vi "Get Item Property Pack Variant.vi"(6 "Default Value":variant, 8 "error in (no error)":errorcluster, 10 "Property Name":string, 11 "CDBase":refnum<k39>) -> (0 "error out":errorcluster, 1 "Found?":bool, 2 "Variant":variant, 3 "CDBase":refnum<k39>)   [LabVIEW 2026, in "Custom Devices Storage.lvlib"]
uses:
  Custom Devices Storage.lvlib
  C:/Users/Administrator/Desktop/Jatin/All DNC DLLs/NationalInstruments.VeriStand.SystemDefinitionAPI.dll
  Jatin/All DNC DLLs/NationalInstruments.VeriStand.SystemDefinitionAPI.dll
  C:/Users/Administrator/Desktop/Jatin/All DNC DLLs/NationalInstruments.VeriStand.SystemStorage.dll
  Jatin/All DNC DLLs/NationalInstruments.VeriStand.SystemStorage.dll
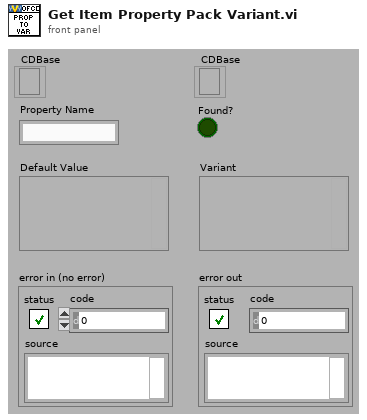
[diagram p1: front panel]
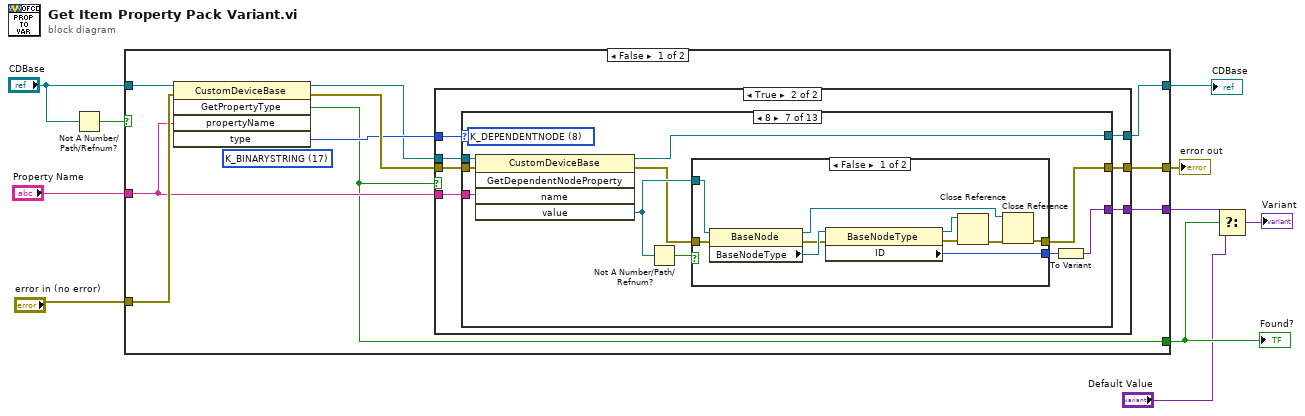
[diagram p0: block diagram]
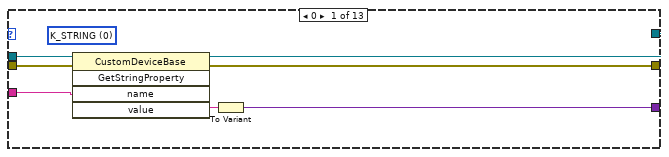
[diagram p3: hidden frame]
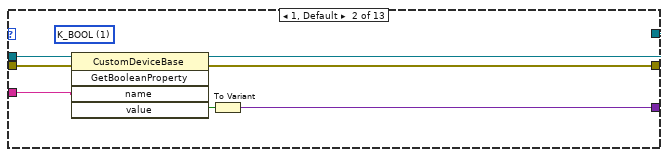
[diagram p4: hidden frame]
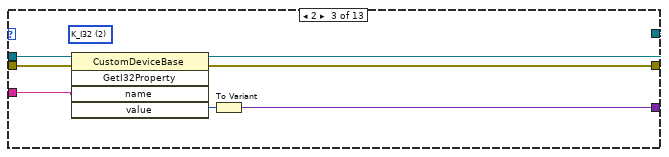
[diagram p5: hidden frame]
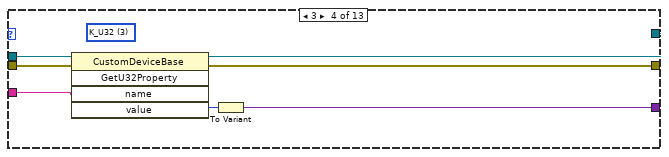
[diagram p6: hidden frame]
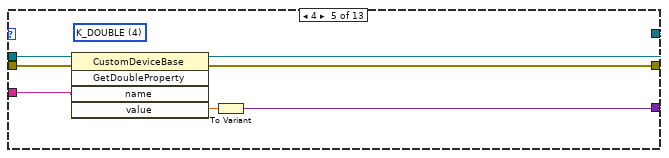
[diagram p7: hidden frame]
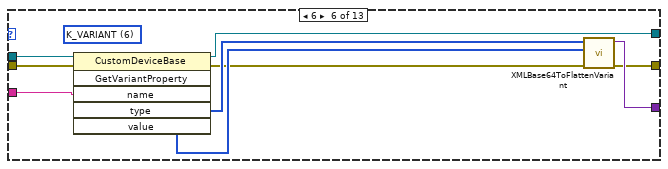
[diagram p8: hidden frame]
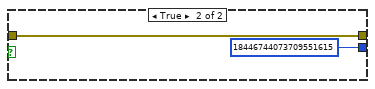
[diagram p9: hidden frame]
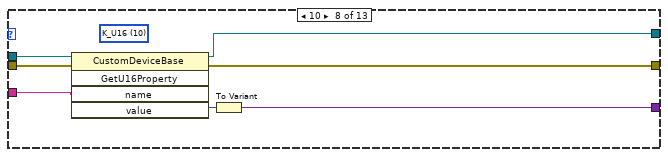
[diagram p10: hidden frame]
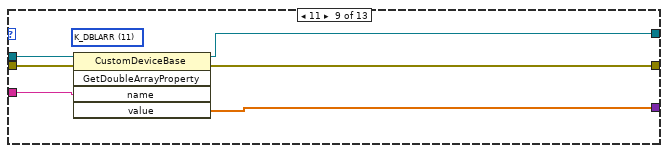
[diagram p11: hidden frame]
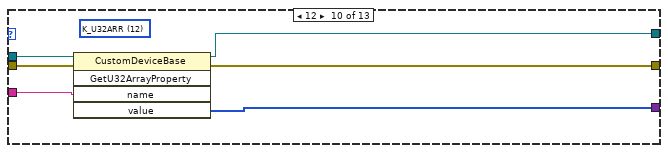
[diagram p12: hidden frame]
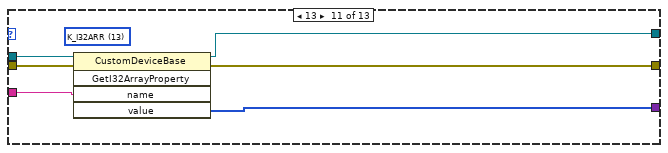
[diagram p13: hidden frame]
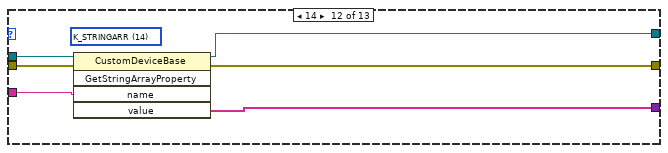
[diagram p14: hidden frame]
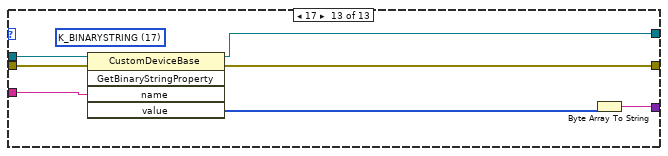
[diagram p15: hidden frame]
diagram:
  n1 = Not A Number/Path/Refnum?(number/path/refnum="CDBase") -> (NaN/Path/Refnum?=w10:bool)
  n2 = case shown="False" w10 {
    tunnel: "Property Name" -> [w15 _]
    tunnel: "CDBase" -> [w20 w135]
    tunnel: "error in (no error)" -> [w19 w134]
    tunnel: [w14 _] -> w6
    tunnel: [w13 _] -> w5
    tunnel: [w12 w135] -> w2
    tunnel: [w11 w134] -> w1
    frame False {
      (unwired) 17 items=["K_STRING", "K_BOOL", "K_I32", "K_U32", "K_DOUBLE", "K_U64", "K_VARIANT", "K_DEPENDENTFILE", "K_DEPENDENTNODE", "K_DATASOURCENODE", "K_U16", "K_DBLARR", "K_U32ARR", "K_I32ARR", "K_STRINGARR", "K_DICTIONARY", "K_DICTIONARYARR", "K_BINARYSTRING"] ("type")
      n3 = invoke class="CustomDeviceBase" method="GetPropertyType"(reference=w20, error in=w19, "propertyName"=w15) -> (reference out=w16:refnum<k39>, error out=w18:errorcluster, "GetPropertyType"=w14:bool, "type"=w17:i32)  [unwired: 2 in, 1 out]
      n4 = case shown="True" w14 {
        tunnel: [w21 w29] -> w12
        tunnel: [w22 w28] -> w11
        tunnel: [_ w27] -> w13
        tunnel: w18 -> [w22 w26]
        tunnel: w17 -> [_ w25]
        tunnel: w16 -> [w21 w24]
        tunnel: w15 -> [_ w23]
        frame False {
        }
        frame True {
          n5 = case shown="8" w25 {
            tunnel: [w36 w43 w50 w57 w64 w73 w80 w102 w108 w114 w120 w122 w127] -> w29
            tunnel: w26 -> [w35 w42 w49 w56 w63 w72 w83 w101 w107 w113 w119 w126 w132]
            tunnel: [w34 w41 w48 w55 w62 w65 w75 w100 w106 w112 w118 w125 w128] -> w28
            tunnel: [w32 w39 w46 w53 w60 w66 w79 w98 w105 w111 w117 w124 w129] -> w27
            tunnel: w24 -> [w30 w38 w44 w51 w58 w71 w82 w97 w103 w110 w116 w121 w133]
            tunnel: w23 -> [w31 w37 w45 w52 w59 w70 w81 w96 w104 w109 w115 w123 w131]
            frame 0 {
              (unwired) 0 items=["K_STRING", "K_BOOL", "K_I32", "K_U32", "K_DOUBLE", "K_U64", "K_VARIANT", "K_DEPENDENTFILE", "K_DEPENDENTNODE", "K_DATASOURCENODE", "K_U16", "K_DBLARR", "K_U32ARR", "K_I32ARR", "K_STRINGARR", "K_DICTIONARY", "K_DICTIONARYARR"] ("type")
              n6 = invoke class="CustomDeviceBase" method="GetStringProperty"(reference=w30, error in=w35, "name"=w31) -> (reference out=w36:refnum<k39>, error out=w34:errorcluster, "value"=w33:string)  [unwired: 2 in, 2 out]
              n7 = To Variant(anything=w33) -> (Variant=w32:variant)
            }
            frame 1, Default {
              (unwired) 1 items=["K_STRING", "K_BOOL", "K_I32", "K_U32", "K_DOUBLE", "K_U64", "K_VARIANT", "K_DEPENDENTFILE", "K_DEPENDENTNODE", "K_DATASOURCENODE", "K_U16", "K_DBLARR", "K_U32ARR", "K_I32ARR", "K_STRINGARR", "K_DICTIONARY", "K_DICTIONARYARR"] ("type")
              n8 = invoke class="CustomDeviceBase" method="GetBooleanProperty"(reference=w38, error in=w42, "name"=w37) -> (reference out=w43:refnum<k39>, error out=w41:errorcluster, "value"=w40:bool)  [unwired: 2 in, 2 out]
              n9 = To Variant(anything=w40) -> (Variant=w39:variant)
            }
            frame 2 {
              (unwired) 2 items=["K_STRING", "K_BOOL", "K_I32", "K_U32", "K_DOUBLE", "K_U64", "K_VARIANT", "K_DEPENDENTFILE", "K_DEPENDENTNODE", "K_DATASOURCENODE", "K_U16", "K_DBLARR", "K_U32ARR", "K_I32ARR", "K_STRINGARR", "K_DICTIONARY", "K_DICTIONARYARR"] ("type")
              n10 = invoke class="CustomDeviceBase" method="GetI32Property"(reference=w44, error in=w49, "name"=w45) -> (reference out=w50:refnum<k39>, error out=w48:errorcluster, "value"=w47:i32)  [unwired: 2 in, 2 out]
              n11 = To Variant(anything=w47) -> (Variant=w46:variant)
            }
            frame 3 {
              (unwired) 3 items=["K_STRING", "K_BOOL", "K_I32", "K_U32", "K_DOUBLE", "K_U64", "K_VARIANT", "K_DEPENDENTFILE", "K_DEPENDENTNODE", "K_DATASOURCENODE", "K_U16", "K_DBLARR", "K_U32ARR", "K_I32ARR", "K_STRINGARR", "K_DICTIONARY", "K_DICTIONARYARR"] ("type")
              n12 = invoke class="CustomDeviceBase" method="GetU32Property"(reference=w51, error in=w56, "name"=w52) -> (reference out=w57:refnum<k39>, error out=w55:errorcluster, "value"=w54:u32)  [unwired: 2 in, 2 out]
              n13 = To Variant(anything=w54) -> (Variant=w53:variant)
            }
            frame 4 {
              (unwired) 4 items=["K_STRING", "K_BOOL", "K_I32", "K_U32", "K_DOUBLE", "K_U64", "K_VARIANT", "K_DEPENDENTFILE", "K_DEPENDENTNODE", "K_DATASOURCENODE", "K_U16", "K_DBLARR", "K_U32ARR", "K_I32ARR", "K_STRINGARR", "K_DICTIONARY", "K_DICTIONARYARR"] ("type")
              n14 = invoke class="CustomDeviceBase" method="GetDoubleProperty"(reference=w58, error in=w63, "name"=w59) -> (reference out=w64:refnum<k39>, error out=w62:errorcluster, "value"=w61:dbl)  [unwired: 2 in, 2 out]
              n15 = To Variant(anything=w61) -> (Variant=w60:variant)
            }
            frame 6 {
              (unwired) 6 items=["K_STRING", "K_BOOL", "K_I32", "K_U32", "K_DOUBLE", "K_U64", "K_VARIANT", "K_DEPENDENTFILE", "K_DEPENDENTNODE", "K_DATASOURCENODE", "K_U16", "K_DBLARR", "K_U32ARR", "K_I32ARR", "K_STRINGARR", "K_DICTIONARY", "K_DICTIONARYARR"] ("type")
              n16 = invoke class="CustomDeviceBase" method="GetVariantProperty"(reference=w71, error in=w72, "name"=w70) -> (reference out=w73:refnum<k39>, error out=w67:errorcluster, "type"=w69:u8[], "value"=w68:u8[])  [unwired: 3 in, 2 out]
              n17 = call "XMLBase64ToFlattenVariant.vi"("error in (no error)"=w67, "Data"=w68, "Type array"=w69) -> ("error out"=w65:errorcluster, "Variant"=w66:variant)  [unwired: 7 in]
            }
            frame 8 {
              (unwired) 8 items=["K_STRING", "K_BOOL", "K_I32", "K_U32", "K_DOUBLE", "K_U64", "K_VARIANT", "K_DEPENDENTFILE", "K_DEPENDENTNODE", "K_DATASOURCENODE", "K_U16", "K_DBLARR", "K_U32ARR", "K_I32ARR", "K_STRINGARR", "K_DICTIONARY", "K_DICTIONARYARR"] ("type")
              n18 = invoke class="CustomDeviceBase" method="GetDependentNodeProperty"(reference=w82, error in=w83, "name"=w81) -> (reference out=w80:refnum<k39>, error out=w76:errorcluster, "value"=w77:refnum<k39>)  [unwired: 2 in, 2 out]
              n19 = Not A Number/Path/Refnum?(number/path/refnum=w77) -> (NaN/Path/Refnum?=w78:bool)
              n20 = case shown="False" w78 {
                tunnel: w76 -> [w93 w95]
                tunnel: [w87 w95] -> w75
                tunnel: w77 -> [w92 _]
                tunnel: [w90 u64 18446744073709551615 ("NodePtr")] -> w74
                frame False {
                  n21 = property class="BaseNode"(reference=w92, error in=w93) -> (reference out=w85:refnum<k39>, error out=w84:errorcluster, "BaseNodeType"=w91:refnum<k39>)
                  n22 = property class="BaseNodeType"(reference=w91, error in=w84) -> (reference out=w86:refnum<k39>, error out=w89:errorcluster, "ID"=w90:u64)
                  n23 = Close Reference(reference=w86, error in (no error)=w89) -> (error out=w88:errorcluster)
                  n24 = Close Reference(reference=w85, error in (no error)=w88) -> (error out=w87:errorcluster)
                }
                frame True {
                }
              }
              n25 = To Variant(anything=w74) -> (Variant=w79:variant)
            }
            frame 10 {
              (unwired) 10 items=["K_STRING", "K_BOOL", "K_I32", "K_U32", "K_DOUBLE", "K_U64", "K_VARIANT", "K_DEPENDENTFILE", "K_DEPENDENTNODE", "K_DATASOURCENODE", "K_U16", "K_DBLARR", "K_U32ARR", "K_I32ARR", "K_STRINGARR", "K_DICTIONARY", "K_DICTIONARYARR"] ("type")
              n26 = invoke class="CustomDeviceBase" method="GetU16Property"(reference=w97, error in=w101, "name"=w96) -> (reference out=w102:refnum<k39>, error out=w100:errorcluster, "value"=w99:u16)  [unwired: 2 in, 2 out]
              n27 = To Variant(anything=w99) -> (Variant=w98:variant)
            }
            frame 11 {
              (unwired) 11 items=["K_STRING", "K_BOOL", "K_I32", "K_U32", "K_DOUBLE", "K_U64", "K_VARIANT", "K_DEPENDENTFILE", "K_DEPENDENTNODE", "K_DATASOURCENODE", "K_U16", "K_DBLARR", "K_U32ARR", "K_I32ARR", "K_STRINGARR", "K_DICTIONARY", "K_DICTIONARYARR"] ("type")
              n28 = invoke class="CustomDeviceBase" method="GetDoubleArrayProperty"(reference=w103, error in=w107, "name"=w104) -> (reference out=w108:refnum<k39>, error out=w106:errorcluster, "value"=w105:dbl[])  [unwired: 2 in, 2 out]
            }
            frame 12 {
              (unwired) 12 items=["K_STRING", "K_BOOL", "K_I32", "K_U32", "K_DOUBLE", "K_U64", "K_VARIANT", "K_DEPENDENTFILE", "K_DEPENDENTNODE", "K_DATASOURCENODE", "K_U16", "K_DBLARR", "K_U32ARR", "K_I32ARR", "K_STRINGARR", "K_DICTIONARY", "K_DICTIONARYARR"] ("type")
              n29 = invoke class="CustomDeviceBase" method="GetU32ArrayProperty"(reference=w110, error in=w113, "name"=w109) -> (reference out=w114:refnum<k39>, error out=w112:errorcluster, "value"=w111:u32[])  [unwired: 2 in, 2 out]
            }
            frame 13 {
              (unwired) 13 items=["K_STRING", "K_BOOL", "K_I32", "K_U32", "K_DOUBLE", "K_U64", "K_VARIANT", "K_DEPENDENTFILE", "K_DEPENDENTNODE", "K_DATASOURCENODE", "K_U16", "K_DBLARR", "K_U32ARR", "K_I32ARR", "K_STRINGARR", "K_DICTIONARY", "K_DICTIONARYARR"] ("type")
              n30 = invoke class="CustomDeviceBase" method="GetI32ArrayProperty"(reference=w116, error in=w119, "name"=w115) -> (reference out=w120:refnum<k39>, error out=w118:errorcluster, "value"=w117:i32[])  [unwired: 2 in, 2 out]
            }
            frame 14 {
              (unwired) 14 items=["K_STRING", "K_BOOL", "K_I32", "K_U32", "K_DOUBLE", "K_U64", "K_VARIANT", "K_DEPENDENTFILE", "K_DEPENDENTNODE", "K_DATASOURCENODE", "K_U16", "K_DBLARR", "K_U32ARR", "K_I32ARR", "K_STRINGARR", "K_DICTIONARY", "K_DICTIONARYARR"] ("type")
              n31 = invoke class="CustomDeviceBase" method="GetStringArrayProperty"(reference=w121, error in=w126, "name"=w123) -> (reference out=w122:refnum<k39>, error out=w125:errorcluster, "value"=w124:string[])  [unwired: 2 in, 2 out]
            }
            frame 17 {
              (unwired) 17 items=["K_STRING", "K_BOOL", "K_I32", "K_U32", "K_DOUBLE", "K_U64", "K_VARIANT", "K_DEPENDENTFILE", "K_DEPENDENTNODE", "K_DATASOURCENODE", "K_U16", "K_DBLARR", "K_U32ARR", "K_I32ARR", "K_STRINGARR", "K_DICTIONARY", "K_DICTIONARYARR", "K_BINARYSTRING"] ("type")
              n32 = invoke class="CustomDeviceBase" method="GetBinaryStringProperty"(reference=w133, error in=w132, "name"=w131) -> (reference out=w127:refnum<k39>, error out=w128:errorcluster, "value"=w130:u8[])  [unwired: 2 in, 2 out]
              n33 = Byte Array To String(unsigned byte array=w130) -> (string=w129:string)
            }
          }
        }
      }
    }
    frame True {
    }
  }
  "CDBase" <- w2
  "Found?" <- w6
  "error out" <- w1
  n34 = Select(t=w5, s=w6, f="Default Value") -> (s? t:f=→"Variant":variant)
